vi "Split FF Infov1.vi"(4 "Team Color Info":T2={"Pink First"=TRUE, "Friend Colors"=enum."Pink over Green"}, 6 "Find Foe":bool=TRUE, 7 "Target":T3={"Rectangle"={"Left"=0, "Top"=0, "Right"=0, "Bottom"=0}, "Area %"=0.0, "FF"=enum."SoF", "Measurements"=[]}) -> (0 "Designation":enum16{"Friend", "Foe"}(ring), 2 "Found":bool, 3 "Target out":T1)   [LabVIEW 2013]
uses:
  Single Target Infov1.ctl
  Team Designationv1.ctl
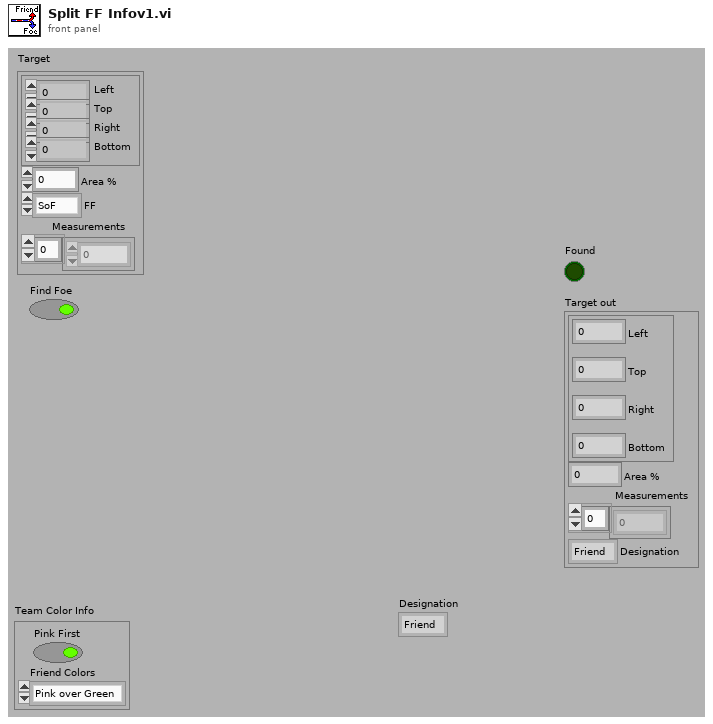
[diagram p1: front panel]
types:
  T1 = cluster{"Rectangle":cluster{"Left":i32, "Top":i32, "Right":i32, "Bottom":i32}, "Area %":dbl, "Measurements":dbl[], "Designation":enum16{"Friend", "Foe"}}
  T2 = cluster{"Pink First":bool, "Friend Colors":enum32{"Pink over Green", "Green over Pink"}}
  T3 = typedef "Single Target Infov1.ctl" = cluster{"Rectangle":cluster{"Left":i32, "Top":i32, "Right":i32, "Bottom":i32}, "Area %":dbl, "FF":T4, "Measurements":dbl[]}
  T4 = typedef "Team Designationv1.ctl" = enum16{"FoS", "SoF"}
  T5 = cluster{"Rectangle":cluster{"Left":i32, "Top":i32, "Right":i32, "Bottom":i32}, "Area %":dbl, "Measurements":dbl[], enum16{"Friend", "Foe"}}
  T6 = cluster{"Left":i32, "Top":i32, "Right":i32, "Bottom":i32}
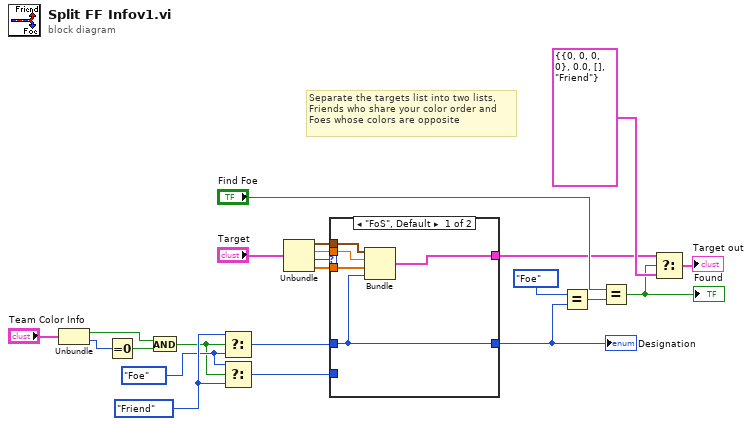
[diagram p0: block diagram]
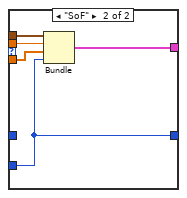
[diagram p2: hidden frame]
diagram:
  w18 = enum16{"Friend", "Foe"}."Foe"
  w19 = enum16{"Friend", "Foe"}."Friend"
  # "Separate the targets list into two lists,\nFriends who share your color order and\nFoes whose colors are opposite"
  n1 = Unbundle("Team Color Info") -> ("Pink First"=w11:bool, "Friend Colors"=w10:enum32{"Pink over Green", "Green over Pink"})
  n2 = Equal To 0?(x=w10) -> (x = 0?=w21:bool)
  n3 = And(x=w11, y=w21) -> (x .and. y?=w16:bool)
  n4 = Select(t=w19, s=w16, f=w18) -> (s? t:f=w20:enum16{"Friend", "Foe"})
  n5 = Select(t=w18, s=w16, f=w19) -> (s? t:f=w17:enum16{"Friend", "Foe"})
  n6 = Unbundle("Target") -> ("Rectangle"=w14:T6, "Area %"=w13:dbl, "FF"=w15:T4, "Measurements"=w9:dbl[])
  n7 = case shown="\"FoS\", Default" w15 {
    tunnel: w14 -> [w27 w32]
    tunnel: w13 -> [w26 w31]
    tunnel: w20 -> [w25 _]
    tunnel: w17 -> [_ w30]
    tunnel: [w25 w30] -> w7
    tunnel: w9 -> [w24 w29]
    tunnel: [w23 w28] -> w3
    frame "FoS", Default {
      n8 = Bundle("Rectangle"=w27, "Area %"=w26, "Measurements"=w24, w25) -> (w23:T5)  [unwired: 1 out]
    }
    frame "SoF" {
      n9 = Bundle("Rectangle"=w32, "Area %"=w31, "Measurements"=w29, w30) -> (w28:T5)  [unwired: 1 out]
    }
  }
  "Designation" <- w7
  n10 = Equal?(x=enum16{"Friend", "Foe"}."Foe", y=w7) -> (x = y?=w6:bool)
  n11 = Equal?(x="Find Foe", y=w6) -> (x = y?=w2:bool)
  "Found" <- w2
  n12 = Select(t=w3, s=w2, f=T5 {"Rectangle"={"Left"=0, "Top"=0, "Right"=0, "Bottom"=0}, "Area %"=0.0, "Measurements"=[], enum."Friend"}) -> (s? t:f=→"Target out":T5)
